vi "RT_PumpMeas_Main.vi"() -> ()   [LabVIEW 2020]
uses:
  <vilib>/NI/STM/SubVIs/MetaDataElement.ctl
  <vilib>/NI/STM/TCP/TCP Write Options.ctl
  TypeDefs/STMLoopState_enum.ctl
  <vilib>/Platform/TimedLoop/XDataNode/timing_clust.ctl
  <vilib>/Platform/TimedLoop/XDataNode/nitl_modes.ctl
  <vilib>/Platform/TimedLoop/XDataNode/wakeup.ctl
  <vilib>/NI/STM/TCP/TCP Read Options.ctl
  PC/PumpMeas/TypeDefs/AIloopTimes.ctl
  Components_global/Queues/InterProcessQueueCtl.ctl
  <vilib>/Utility/error.llb/DialogType.ctl
  <vilib>/NI/STM/TCP/Write Meta Data (TCP Ref).vi
  <vilib>/NI/STM/TCP/Get Connection Reference (TCP).vi
  <vilib>/NI/STM/TCP/Write Meta Data (TCP Clst).vi
  <vilib>/FPGAPlugInAG/cRIO-9064/niLvFpga_Open_cRIO-9064.vi
  <vilib>/rvi/interface/common/dynamic/niFpgaDynamicAddResources.vi
  <vilib>/Utility/error.llb/Error Cluster From Error Code.vi
  <vilib>/rvi/errors/niLvFpgaAdjustHostInterfaceError.vi
  <vilib>/NI/STM/TCP/Write Message (TCP).vi
  <vilib>/NI/STM/TCP/Read Message (TCP).vi
  <vilib>/FPGAPlugInAG/Dynamic/niLvFpga_Close_Dynamic.vi
  <vilib>/rvi/interface/nirviOpenFPGA/nirviOpenFPGA.xnode
  FPGA Bitfiles/pumpmeasurements_FPGATarget2_FPGAmain_ubfhyL6MIb0.lvbitx
  <vilib>/Platform/TimedLoop/XDataNode/XDataNode.xnode
  <vilib>/rvi/interface/nirviReadWriteControl/nirviReadWriteControl.xnode
  <vilib>/rvi/interface/nirviCloseFPGA/nirviCloseFPGA.xnode
  <vilib>/NI/STM/NI STM.lvlib
  Components_global/Timing/Timing.lvlib
  <vilib>/Platform/TimedLoop/XDataNode/XDNodeRunTimeDep.lvlib
  Components_global/Queues/Queues.lvlib
  <vilib>/rvi/interface/Simulation/niFpgaSimulationCallBeginRW.vi
  NiFpgaLv.dll
panel:
  out "Ts [ms] 2":dbl caption="NI9208 AI Loop \nTime (Ts) [ms]"
  out "Ts [ms]":dbl caption="NI9205 AI Loop \nTime (Ts) [ms]"
  out "ReadLoop FinishedLate Counter":dbl
  out "ReadLoop Iteration \nDuration (us)":i64
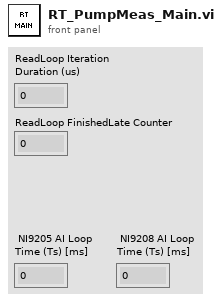
[diagram p1: front panel]
types:
  T1 = typedef "STMLoopState_enum.ctl" = enum16{"Initialize", "Warm-up", "Run", "ShutDown"}
  T2 = typedef "NI STM.lvlib/TCP Write Options.ctl" = cluster{"ignore timeout error":bool, "timeout ms (1000)":i32}
  T3 = typedef "NI STM.lvlib/MetaDataElement.ctl" = string
  T4 = typedef "NI STM.lvlib/TCP Connection Info.ctl" = cluster{"connection ID":refnum<k5>, "meta data":T3[]}
  T5 = typedef "Queues.lvlib/Queue Refs.ctl" = cluster{"InterProcessQueue":refnum<queue>}
  T6 = typedef "XDNodeRunTimeDep.lvlib/timing_clust.ctl" = cluster{"Expected End [f-1]":u64, "Actual End [f-1]":u64, "Finished Late? [f-1]":bool, "Expected End [i-1]":u64, "Actual End [i-1]":u64, "Finished Late? [i-1]":bool, "Expected Start [i]":u64, "Actual Start [i]":u64, "Expected Start [f]":u64, "Actual Start [f]":u64, "Source Name":string, "Structure Name":string, "Period":i64, "Deadline":i64, "Offset":i64, "Start":i64, "Priority":i32, "Timeout":i32, "Mode":T7, "Wakeup Reason":T8, "Error":errorcluster, "Source Type":string, "Secondary Source Type":string, "Global End Time":u64, "Global Start Time":u64, "Frame Duration":u64, "Iteration Duration":u64, "Assigned CPU":i32, "I/O Scan Engine Mode":u32}
  T7 = typedef "XDNodeRunTimeDep.lvlib/nitl_modes.ctl" = enum32{"No Change", "Process missed periods, maintain original phase", "Discard missed periods, maintain original phase", "Process missed periods, ignore original phase", "Discard missed periods, ignore original phase"}
  T8 = typedef "XDNodeRunTimeDep.lvlib/wakeup.ctl" = enum32{"Normal", "Aborted", "Asynchronous wakeup", "Timing source error", "Timed loop error", "Timeout"}
  T9 = typedef "NI STM.lvlib/TCP Read Options.ctl" = cluster{"ignore timeout error":bool, "timeout ms (1000)":i32}
  T10 = typedef "AIloopTimes.ctl" = cluster{"NI 9205 loop time":dbl, "NI 9208 loop time":dbl}
  T11 = typedef "Queues.lvlib/InterProcessQueueCtl.ctl" = cluster{"Command":string, "Data":variant}
  T12 = typedef "DialogType.ctl" = u16
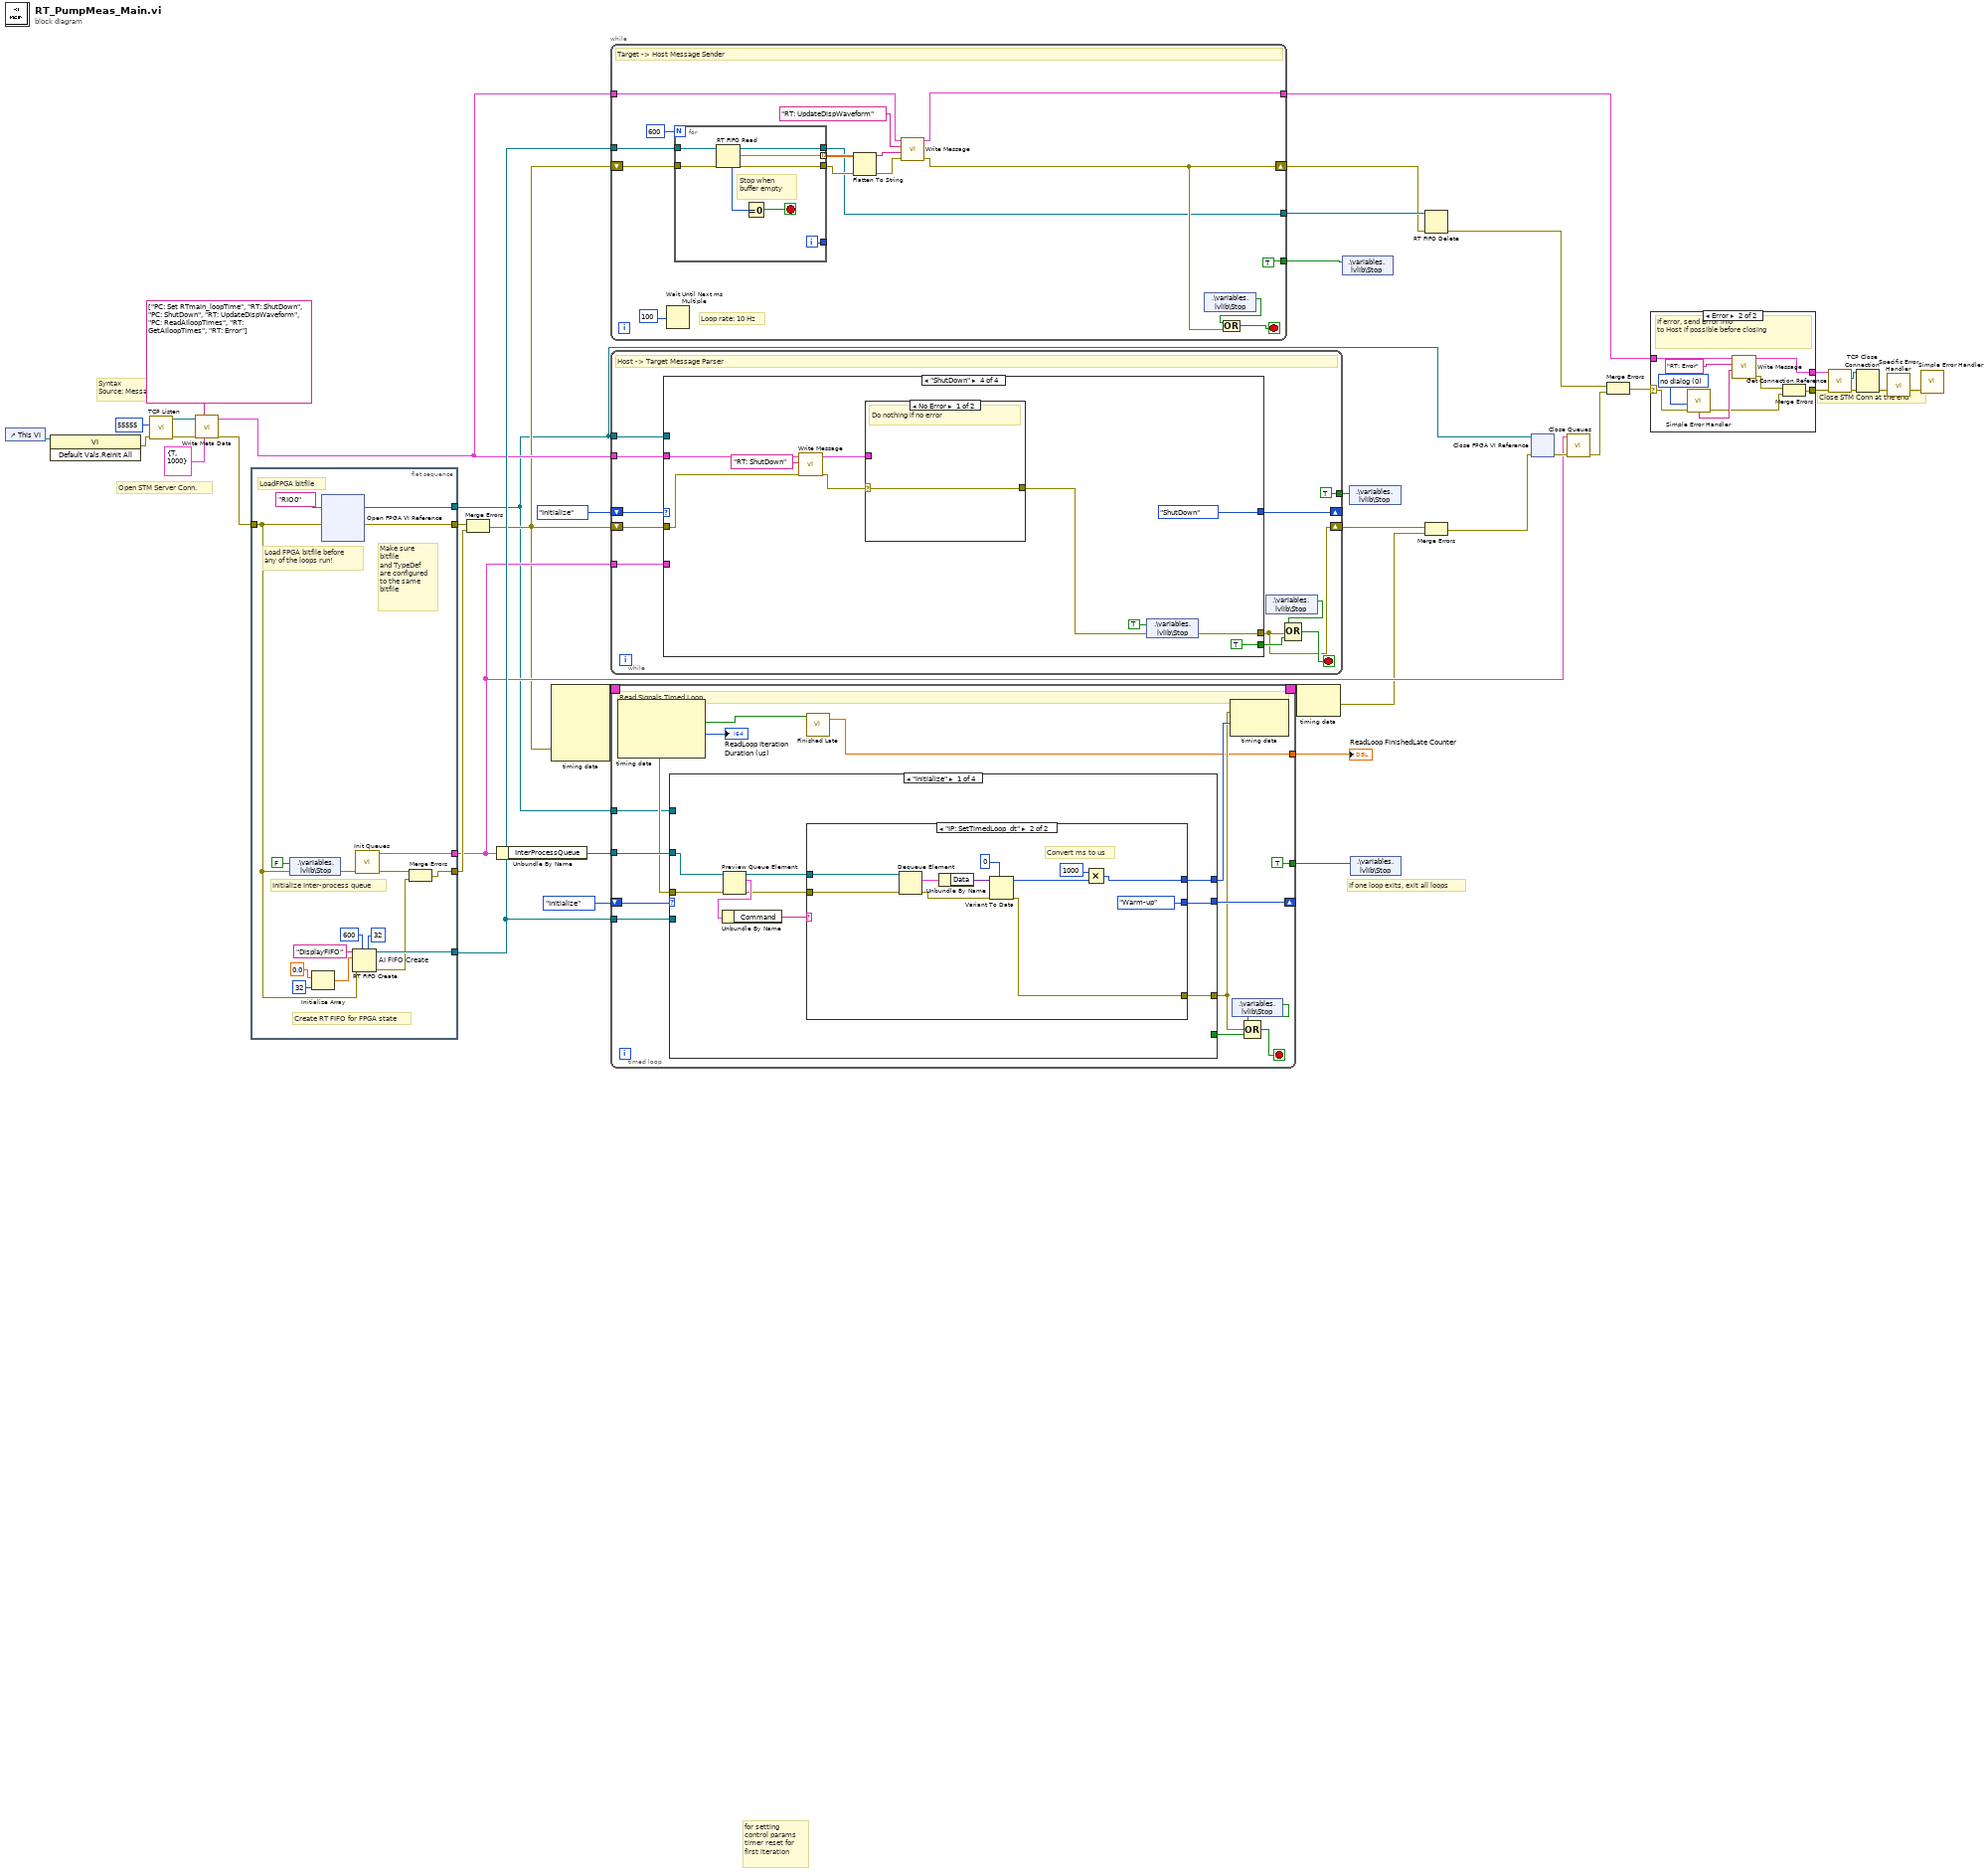
[diagram p0: block diagram]
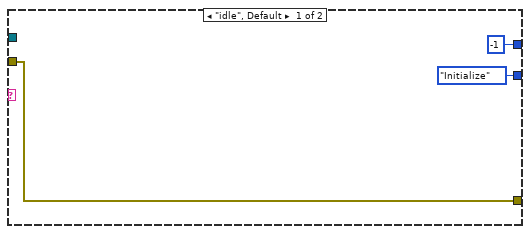
[diagram p2: hidden frame]
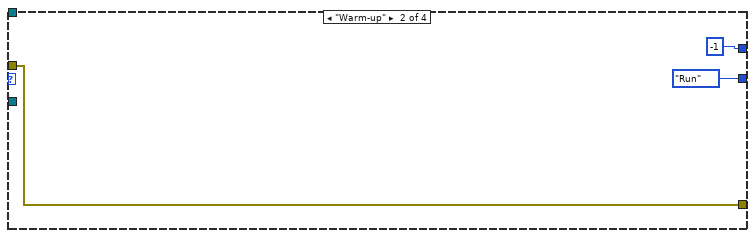
[diagram p3: hidden frame]
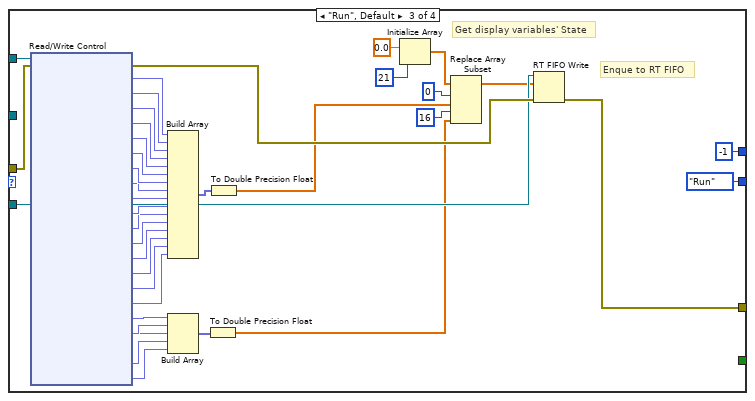
[diagram p4: hidden frame]
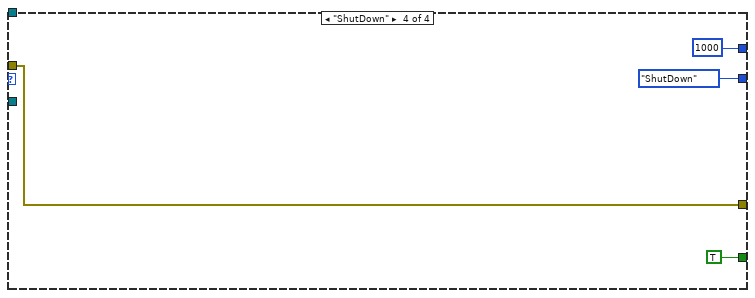
[diagram p5: hidden frame]
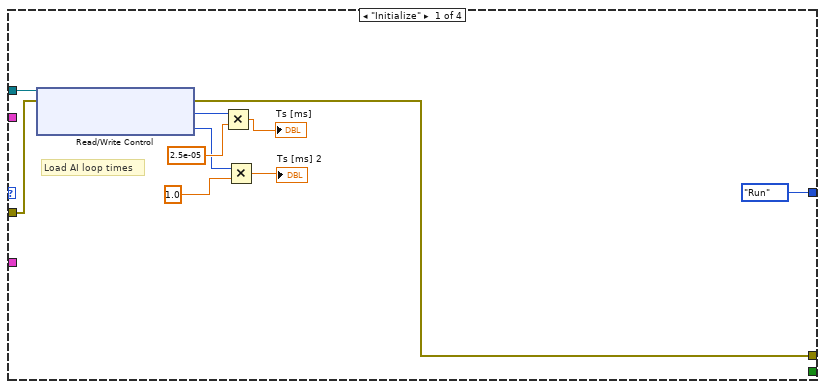
[diagram p6: hidden frame]
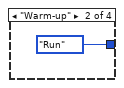
[diagram p7: hidden frame]
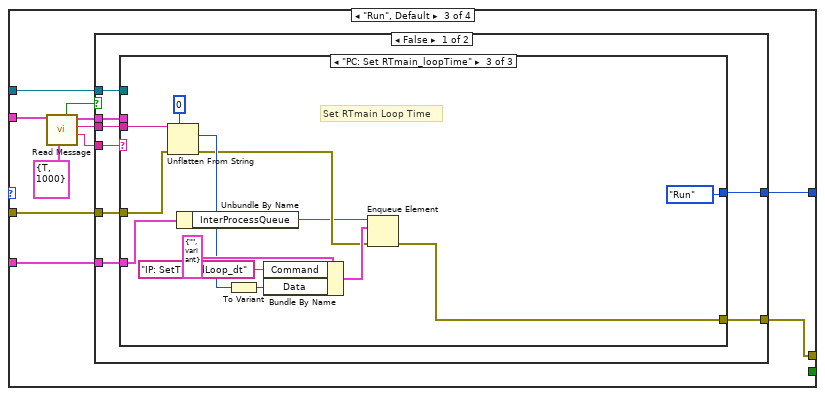
[diagram p8: hidden frame]
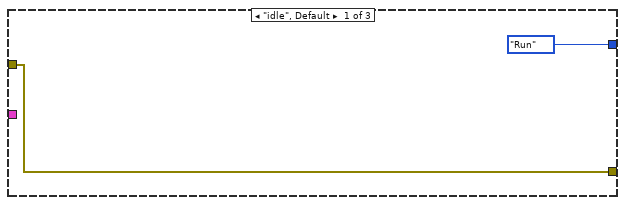
[diagram p9: hidden frame]
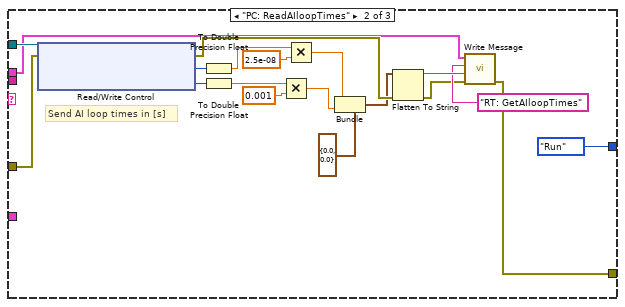
[diagram p10: hidden frame]
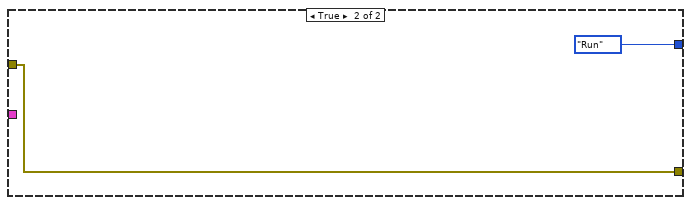
[diagram p11: hidden frame]
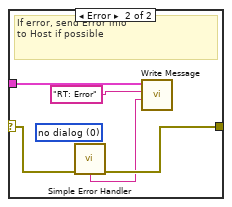
[diagram p12: hidden frame]
diagram:
  # "for setting control params\ntimer reset for\nfirst iteration"
  # "Close STM Conn at the end"
  # "Syntax\nSource: Message"
  # "Open STM Server Conn."
  # "If one loop exits, exit all loops"
  n1 = control-ref of="This VI"() -> (w9:refnum<vi>)
  n2 = invoke on="Invoke Node" class="VI" method="Default Vals.Reinit All"(reference=w9) -> (error out=w8:errorcluster)  [unwired: 2 in, 2 out]
  n3 = call <vilib>:"TCP Listen.vi"("error in (no error)"=w8, "port"=u16 55555) -> ("error out"=w39:errorcluster, "connection ID"=w38:refnum<k5>)  [unwired: 5 in, 3 out]
  n4 = call-poly <vilib>:"Write Meta Data.vi"("options"=T2 {"ignore timeout error"=TRUE, "timeout ms (1000)"=1000}, "meta data"=T3[] ["PC: Set RTmain_loopTime", "RT: ShutDown", "PC: ShutDown", "RT: UpdateDispWaveform", "PC: ReadAIloopTimes", "RT: GetAIloopTimes", "RT: Error"], "error in"=w39, "connection ID"=w38) -> ("error out"=w34:errorcluster, "connection info out"=w7:T4)  [unwired: 1 in, 5 out]
  n5 = flat-sequence {
    tunnel: w34 -> [w42]
    tunnel: [w41] -> w1
    tunnel: [w57] -> w30
    tunnel: [w55] -> w5
    tunnel: [w45] -> w29
    tunnel: [w48] -> w25
    frame #0 {
      # "Make sure \nbitfile \nand TypeDef \nare configured\nto the same \nbitfile"
      # "Create RT FIFO for FPGA state"
      # "LoadFPGA bitfile"
      # "Initialize Inter-process queue"
      # "Load FPGA bitfile before \nany of the loops run!"
      n6 = shared-variable ".\\variables.lvlib\\Stop"(FALSE ("Stop"), error in=w42) -> (error out=w47:errorcluster)
      n7 = Initialize Array(0.0 ("element"), 32 ("dimension size")) -> (w50:dbl[])
      n8 = xnode "Open FPGA VI Reference"("error in"=w42, "resource name"=tag "RIO0") -> ("FPGA VI Reference Out"=w41:refnum<k20>, "error out"=w57:errorcluster)
      n9 = RT FIFO Create "AI FIFO Create"(0:"DisplayFIFO" ("name (unnamed)"), 1:w50, 3:w42, 4:u32 600 ("size (10)"), 6:u32 32 ("elements in array (1)")) -> (8:w48:refnum<k33>, 11:w43:errorcluster)  [unwired: 3 in, 1 out]
      n10 = call "Init Queues.vi"("error in (no error)"=w47) -> ("error out"=w44:errorcluster, "Queue Refs"=w55:T5)  [unwired: 9 in]
      n11 = Merge Errors(w44, w43) -> (w45:errorcluster)
    }
  }
  n12 = Merge Errors(w30, w29) -> (w2:errorcluster)
  n13 = Unbundle By Name(w5) -> ("InterProcessQueue"=w28:refnum<queue>)
  n14 = node-c288(w2) -> (w33:T6)  [unwired: 4 in]
  n15 = timed-loop {
    timing: w33 -> [_]
    timing-out: [_] -> w32
    shift-right: [w71] -> _
    shift-left: STMLoopState_enum."Initialize" ("RTmainLoopState") -> [w72]
    tunnel: w28 -> [w68]
    tunnel: [TRUE ("Stop")] -> w27
    tunnel: w25 -> [w60]
    tunnel: w1 -> [w59]
    tunnel: [w58] -> w12
    stop <- w65 stop-if-true
    # "Read Signals Timed Loop"
    n16 = node-c288() -> (w66:errorcluster, w70:bool, →"ReadLoop Iteration \nDuration (us)":i64)  [unwired: 1 in, 1 out]
    n17 = case shown="\"Initialize\"" w72 {
      tunnel: [w78 STMLoopState_enum."Run" ("RTmainLoopState") STMLoopState_enum."Run" ("RTmainLoopState") STMLoopState_enum."ShutDown" ("RTmainLoopState")] -> w71
      tunnel: [_ _ _ TRUE] -> w64
      tunnel: w68 -> [w77 _ _ _]
      tunnel: [w76 i64 -1 ("Period") i64 -1 ("Period") i64 1000 ("Period")] -> w67
      tunnel: w66 -> [w75 w96 w133 w137]
      tunnel: [w73 w96 w129 w137] -> w63
      tunnel: w60 -> [_ _ w128 _]
      tunnel: w59 -> [_ _ w134 _]
      frame "Initialize" {
        n18 = Preview Queue Element(queue=w77, error in (no error)=w75) -> (queue out=w81:refnum<queue>, element=w80:cluster{"Command":string, "Data":variant}, error out=w74:errorcluster)  [unwired: 1 in, 1 out]
        n19 = Unbundle By Name(w80) -> ("Command"=w79:string)
        n20 = case shown="\"IP: SetTimedLoop_dt\"" w79 {
          tunnel: w81 -> [_ w94]
          tunnel: [STMLoopState_enum."Initialize" ("RTmainLoopState") STMLoopState_enum."Warm-up" ("RTmainLoopState")] -> w78
          tunnel: [i64 -1 w85] -> w76
          tunnel: w74 -> [w82 w90]
          tunnel: [w82 w88] -> w73
          frame "idle", Default {
          }
          frame "IP: SetTimedLoop_dt" {
            # "Convert ms to us"
            n21 = Dequeue Element(queue=w94, error in (no error)=w90) -> (element=w93:cluster{"Command":string, "Data":variant}, error out=w89:errorcluster)  [unwired: 1 in, 2 out]
            n22 = Unbundle By Name(w93) -> ("Data"=w92:variant)
            n23 = Variant To Data(error in=w89, type=i64 0, Variant=w92) -> (data=w86:i64, error out=w88:errorcluster)
            n24 = Multiply(x=i64 1000, y=w86) -> (x*y=w85:i64)
          }
        }
      }
      frame "Warm-up" {
      }
      frame "Run", Default {
        # "Enque to RT FIFO"
        # "Get display variables' State"
        n25 = xnode "Read/Write Control"("FPGA VI Reference In"=w134, "error in"=w133) -> ("error out"=w130:errorcluster, "NI9205: AI0 [V]"=w125:fxp<+/-,35,5>, "NI9205: AI1 [V]"=w124:fxp<+/-,35,5>, "NI9205: AI2 [V]"=w123:fxp<+/-,35,5>, "NI9205: AI3 [V]"=w122:fxp<+/-,35,5>, "NI9205: AI4 [V]"=w121:fxp<+/-,35,5>, "NI9205: AI5 [V]"=w120:fxp<+/-,35,5>, "NI9205: AI6 [V]"=w119:fxp<+/-,35,5>, "NI9205: AI7 [V]"=w118:fxp<+/-,35,5>, "NI9205: AI16 [V]"=w117:fxp<+/-,35,5>, "NI9205: AI17 [V]"=w116:fxp<+/-,35,5>, "NI9205: AI18 [V]"=w115:fxp<+/-,35,5>, "NI9205: AI19 [V]"=w114:fxp<+/-,35,5>, "NI9205: AI20 [V]"=w113:fxp<+/-,35,5>, "NI9205: AI21 [V]"=w112:fxp<+/-,35,5>, "NI9205: AI22 [V]"=w111:fxp<+/-,35,5>, "NI9205: AI23 [V]"=w99:fxp<+/-,35,5>, "NI9208: AI0 [A]"=w110:fxp<+/-,24,-4>, "NI9208: AI1 [A]"=w109:fxp<+/-,24,-4>, "NI9208: AI2 [A]"=w108:fxp<+/-,24,-4>, "NI9208: AI3 [A]"=w107:fxp<+/-,24,-4>, "NI9208: AI4 [A]"=w106:fxp<+/-,24,-4>)  [unwired: 1 out]
        n26 = Build Array(w125, w124, w123, w122, w121, w120, w119, w118, w117, w116, w115, w114, w113, w112, w111, w99) -> (w105:fxp<+/-,35,5>[])
        n27 = Build Array(w110, w109, w108, w107, w106) -> (w103:fxp<+/-,24,-4>[])
        n28 = To Double Precision Float(number=w103) -> (double precision float=w102:dbl[])
        n29 = To Double Precision Float(number=w105) -> (double precision float=w104:dbl[])
        n30 = Initialize Array(0.0 ("element"), 21 ("dimension size")) -> (w127:dbl[])
        n31 = Replace Array Subset(array=w127, new element #1=w104, index #1=0 ("index"), new element #2=w102, index #2=16 ("index")) -> (w126:dbl[])
        n32 = RT FIFO Write(0:w128, 1:w126, 3:w130) -> (11:w129:errorcluster)  [unwired: 2 in, 3 out]
      }
      frame "ShutDown" {
      }
    }
    n33 = call "Finished Late.vi"("Finished \nLate?"=w70) -> ("# Finished\nLate counter"=w58:dbl)  [unwired: 8 in, 2 out]
    n34 = node-c288(w63, w67) -> ()  [unwired: 1 out]
    n35 = shared-variable ".\\variables.lvlib\\Stop"() -> (w61:bool)  [unwired: 1 in, 1 out]
    n36 = Compound Arithmetic op=OR(w61, w63, w64) -> (w65:bool)
  }
  "ReadLoop FinishedLate Counter" <- w12
  n37 = while {
    tunnel: w25 -> [w164]
    tunnel: w7 -> [w161]
    tunnel: [w152] -> w15
    tunnel: [w151] -> w24
    tunnel: [TRUE ("Stop")] -> w11
    shift-right: [w154] -> w18
    shift-left: w2 -> [w149]
    stop <- w153 stop-if-true
    # "Loop rate: 10 Hz"
    # "Target -> Host Message Sender"
    n38 = Wait Until Next ms Multiple(millisecond multiple=u32 100) -> ()  [unwired: 1 out]
    n39 = for {
      N: 600 -> [_]
      tunnel: w164 -> [w172]
      tunnel: [w169] -> w159 mode=indexing
      tunnel: w149 -> [w168]
      tunnel: [w167] -> w157
      tunnel: [w166] -> w151
      tunnel: [w165] -> _
      i -> [w165]
      stop <- w170 stop-if-true
      # "Stop when\nbuffer empty"
      n40 = RT FIFO Read(0:w172, 3:w168) -> (7:w171:u32, 8:w166:refnum<k33>, 9:w169:dbl[], 11:w167:errorcluster)  [unwired: 2 in, 1 out]
      n41 = Equal To 0?(x=w171) -> (x = 0?=w170:bool)
    }
    n42 = Flatten To String(anything=w159, error in (no error)=w157) -> (data string=w158:string, error out=w156:errorcluster)  [unwired: 2 in, 1 out]
    n43 = call-poly <vilib>:"Write Message.vi"("error in"=w156, "data"=w158, "name"="RT: UpdateDispWaveform", "connection info in"=w161) -> ("error out"=w154:errorcluster, "connection info out"=w152:T4)  [unwired: 6 in]
    n44 = shared-variable ".\\variables.lvlib\\Stop"() -> (w155:bool)  [unwired: 1 in, 1 out]
    n45 = Compound Arithmetic op=OR(w155, w154) -> (w153:bool)
  }
  n46 = while {
    shift-right: [w181] -> _
    shift-left: STMLoopState_enum."Initialize" ("RTmainLoopState") -> [w183]
    tunnel: w7 -> [w182]
    tunnel: w1 -> [w178]
    tunnel: w5 -> [w176]
    tunnel: [TRUE ("Stop")] -> w26
    shift-right: [w173] -> w10
    shift-left: w2 -> [w177]
    stop <- w179 stop-if-true
    # "Host -> Target Message Parser"
    n47 = case shown="\"ShutDown\"" w183 {
      tunnel: w182 -> [_ _ w203 w257]
      tunnel: [STMLoopState_enum."Run" ("RTmainLoopState") STMLoopState_enum."Run" ("RTmainLoopState") w197 STMLoopState_enum."ShutDown" ("RTmainLoopState")] -> w181
      tunnel: [_ _ _ TRUE] -> w180
      tunnel: [w189 _ w201 w254] -> w173
      tunnel: w178 -> [w192 _ w202 _]
      tunnel: w177 -> [w191 _ w199 w256]
      tunnel: w176 -> [_ _ w195 _]
      frame "Initialize" {
        # "Load AI loop times"
        n48 = xnode "Read/Write Control"("FPGA VI Reference In"=w192, "error in"=w191) -> ("error out"=w189:errorcluster, "NI9205 AI loop time [ticks]"=w187:u32, "NI9208 AI loop time [ms]"=w185:u32)  [unwired: 1 out]
        n49 = Multiply(x=w187, y=2.5e-05) -> (x*y=→"Ts [ms]":dbl)
        n50 = Multiply(x=w185, y=1.0) -> (x*y=→"Ts [ms] 2":dbl)
      }
      frame "Warm-up" {
      }
      frame "Run", Default {
        n51 = call-poly <vilib>:"Read Message.vi"("options"=T9 {"ignore timeout error"=TRUE, "timeout ms (1000)"=1000}, "connection info in"=w203) -> ("name"=w205:T3, "data string"=w204:string, "connection info out"=w196:T4, "timed out?"=w200:bool)  [unwired: 3 in, 3 out]
        n52 = case shown="False" w200 {
          tunnel: w205 -> [w213 _]
          tunnel: w204 -> [w212 _]
          tunnel: w202 -> [w211 _]
          tunnel: [w210 w248] -> w201
          tunnel: w199 -> [w209 w248]
          tunnel: [w208 STMLoopState_enum."Run" ("RTmainLoopState")] -> w197
          tunnel: w196 -> [w207 _]
          tunnel: w195 -> [w206 _]
          frame False {
            n53 = case shown="\"PC: Set RTmain_loopTime\"" w213 {
              tunnel: w212 -> [_ _ w239]
              tunnel: w211 -> [_ w234 _]
              tunnel: [w215 w225 w235] -> w210
              tunnel: w209 -> [w215 w233 w236]
              tunnel: [STMLoopState_enum."Run" ("RTmainLoopState") STMLoopState_enum."Run" ("RTmainLoopState") STMLoopState_enum."Run" ("RTmainLoopState")] -> w208
              tunnel: w207 -> [_ w228 _]
              tunnel: w206 -> [_ _ w238]
              frame "idle", Default {
              }
              frame "PC: ReadAIloopTimes" {
                # "Send AI loop times in [s]"
                n54 = xnode "Read/Write Control"("FPGA VI Reference In"=w234, "error in"=w233) -> ("error out"=w230:errorcluster, "NI9205 AI loop time [ticks]"=w223:u32, "NI9208 AI loop time [ms]"=w220:u32)  [unwired: 1 out]
                n55 = To Double Precision Float(number=w223) -> (double precision float=w231:dbl)
                n56 = To Double Precision Float(number=w220) -> (double precision float=w222:dbl)
                n57 = Multiply(x=w222, y=0.001) -> (x*y=w218:dbl)
                n58 = Multiply(x=w231, y=2.5e-08) -> (x*y=w219:dbl)
                n59 = Bundle(cluster=T10 {"NI 9205 loop time"=0.0, "NI 9208 loop time"=0.0} ("AI loop times [s]"), "NI 9205 loop time"=w219, "NI 9208 loop time"=w218) -> (w217:T10)
                n60 = Flatten To String(anything=w217, error in (no error)=w230) -> (data string=w229:string, error out=w226:errorcluster)  [unwired: 2 in, 1 out]
                n61 = call-poly <vilib>:"Write Message.vi"("error in"=w226, "data"=w229, "name"="RT: GetAIloopTimes", "connection info in"=w228) -> ("error out"=w225:errorcluster)  [unwired: 6 in, 1 out]
              }
              frame "PC: Set RTmain_loopTime" {
                # "Set RTmain Loop Time"
                n62 = Unflatten From String(type=i64 0 ("Period"), binary string=w239, error in (no error)=w236) -> (value=w244:i64, error out=w241:errorcluster)  [unwired: 2 in, 1 out]
                n63 = Unbundle By Name(w238) -> ("InterProcessQueue"=w237:refnum<queue>)
                n64 = To Variant(anything=w244) -> (Variant=w245:variant)
                n65 = Bundle By Name(cluster=T11 {"Command"="", "Data"=variant} ("STMparseQueue"), "Command"="IP: SetTimedLoop_dt", "Data"=w245) -> (w242:T11)
                n66 = Enqueue Element(queue=w237, element=w242, error in (no error)=w241) -> (error out=w235:errorcluster)  [unwired: 1 in, 2 out]
              }
            }
          }
          frame True {
          }
        }
      }
      frame "ShutDown" {
        n67 = call-poly <vilib>:"Write Message.vi"("error in"=w256, "name"="RT: ShutDown", "connection info in"=w257) -> ("error out"=w252:errorcluster, "connection info out"=w251:T4)  [unwired: 7 in]
        n68 = case shown="No Error" w252 {
          selector: w252 -> [w260 w263]
          tunnel: w251 -> [_ w264]
          tunnel: [w260 w262] -> w250
          frame No Error {
            # "Do nothing if no error"
          }
          frame Error {
            (unwired) T12 0 items=["no dialog", "OK message", "continue or stop message", "OK message + warnings", "continue/stop + warnings"] ("type of dialog (OK msg:1)")
            # "If error, send Error info \nto Host if possible"
            n69 = call <vilib>:"Simple Error Handler.vi"("error in (no error)"=w263) -> ("error out"=w262:errorcluster, "message"=w261:string)  [unwired: 4 in, 3 out]
            n70 = call-poly <vilib>:"Write Message.vi"("data"=w261, "name"="RT: Error", "connection info in"=w264) -> ()  [unwired: 7 in, 2 out]
          }
        }
        n71 = shared-variable ".\\variables.lvlib\\Stop"(TRUE ("Stop"), error in=w250) -> (error out=w254:errorcluster)
      }
    }
    n72 = shared-variable ".\\variables.lvlib\\Stop"() -> (w174:bool)  [unwired: 1 in, 1 out]
    n73 = Compound Arithmetic op=OR(w174, w173, w180) -> (w179:bool)
  }
  n74 = node-c288(w32) -> (w3:errorcluster)
  n75 = shared-variable ".\\variables.lvlib\\Stop"(w11) -> ()  [unwired: 1 in, 1 out]
  n76 = shared-variable ".\\variables.lvlib\\Stop"(w26) -> ()  [unwired: 1 in, 1 out]
  n77 = shared-variable ".\\variables.lvlib\\Stop"(w27) -> ()  [unwired: 1 in, 1 out]
  n78 = RT FIFO Delete(0:w24, 3:w18) -> (11:w23:errorcluster)  [unwired: 1 in]
  n79 = Merge Errors(w10, w3) -> (w17:errorcluster)
  n80 = xnode "Close FPGA VI Reference"("FPGA VI Reference In"=w1, "error in"=w17) -> ("error out"=w6:errorcluster)
  n81 = call "Close Queues.vi"("error in (no error)"=w6, "FIFOs In"=w5) -> ("error out"=w4:errorcluster)  [unwired: 9 in]
  n82 = Merge Errors(w23, w4) -> (w16:errorcluster)
  n83 = case shown="Error" w16 {
    selector: w16 -> [w266 w272]
    tunnel: w15 -> [w267 w275]
    tunnel: [w266 w268] -> w14
    tunnel: [w267 w274] -> w13
    frame No Error {
      # "Do nothing if no error"
    }
    frame Error {
      w273 = T12 0 items=["no dialog", "OK message", "continue or stop message", "OK message + warnings", "continue/stop + warnings"] ("type of dialog (OK msg:1)")
      # "If error, send Error info \nto Host if possible before closing"
      n84 = call <vilib>:"Simple Error Handler.vi"("type of dialog (OK msg:1)"=w273, "error in (no error)"=w272) -> ("error out"=w269:errorcluster, "message"=w271:string)  [unwired: 3 in, 3 out]
      n85 = call-poly <vilib>:"Write Message.vi"("data"=w271, "name"="RT: Error", "connection info in"=w275) -> ("error out"=w270:errorcluster, "connection info out"=w274:T4)  [unwired: 7 in]
      n86 = Merge Errors(w270, w269) -> (w268:errorcluster)
    }
  }
  n87 = call-poly <vilib>:"Get Connection Reference.vi"("error in"=w14, "connection info in"=w13) -> ("error out"=w22:errorcluster, "connection ID out"=w21:refnum<k5>)  [unwired: 7 in, 1 out]
  n88 = TCP Close Connection(connection ID=w21, error in (no error)=w22) -> (error out=w20:errorcluster)  [unwired: 1 in, 1 out]
  n89 = call "Specific Error Handler"("Error to Check"=w20) -> ("error out"=w19:errorcluster)  [unwired: 11 in, 3 out]
  n90 = call <vilib>:"Simple Error Handler.vi"("error in (no error)"=w19) -> ()  [unwired: 4 in, 5 out]
